vi "Layout - Standard.vi"(8 "Error in":errorcluster caption="Error in (no error)", 11 "Content":string) -> (0 "Error out":errorcluster, 3 "Text Output":string)   [LabVIEW 2023, in "Confluence Formatting.lvlib"]
uses:
  Confluence Formatting.lvlib
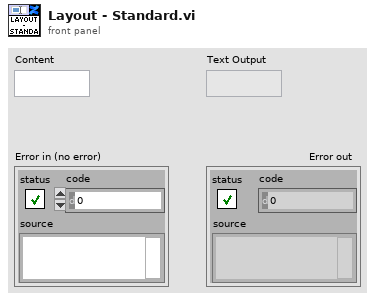
[diagram p1: front panel]
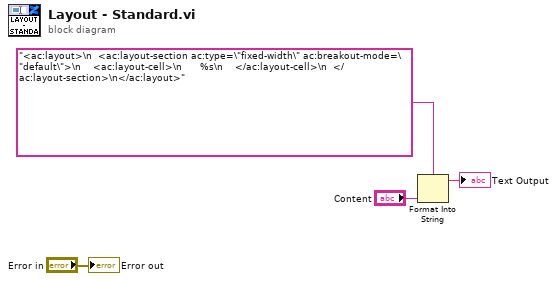
[diagram p0: block diagram]
diagram:
  n1 = Format Into String(format string="<ac:layout>\n  <ac:layout-section ac:type=\"fixed-width\" ac:breakout-mode=\"default\">\n    <ac:layout-cell>\n      %s\n    </ac:layout-cell>\n  </ac:layout-section>\n</ac:layout>", "Content") -> (resulting string=→"Text Output":string)  [unwired: 2 in, 1 out]
  "Error out" <- "Error in"
